vi "PKG_Fill_MUL32A.vi"(1 "dest_axis":i16, 4 "dest":i16, 5 "Src2_axis":i16, 6 "Src2":i16, 7 "Src1_axis":i16, 9 "Src1":i16, 10 "EventType":i16, 11 "info":T1) -> (2 "function return":i32, 3 "info out":T1)   [LabVIEW 2011, in "IMC_Pkg4xxx.lvlib"]
doc: "IMC_PKG_API int WINAPI PKG_Fill_MUL32A(EventInfo *info, short EventType, short Src1, short Src1_axis, short Src2, short Src2_axis, short dest, short dest_axis);\n\n\nIMC_PKG_API int WINAPI PKG_Fill_SCA32(EventInfo *info, short EventType, short Src1, short Src1_axis, short Src2, short Src2_axis, short dest, short dest_axis); IMC_PKG_API int WINAPI PKG_Fill_SCA32i(EventInfo *info, short EventType, short Src1, short Src1_axis, double data, short dest, short dest_axis); IMC_PKG_API int WINAPI PKG_Fill_SCA48(EventInfo *info, short EventType, short Src1, short Src1_axis, short Src2, short Src2_axis, short dest, short dest_axis); IMC_PKG_API int WINAPI PKG_Fill_SCA48i(EventInfo *info, short EventType, short Src1, short Src1_axis, double data, short dest, short dest_axis); IMC_PKG_API int WINAPI PKG_Fill_MUL32L(EventInfo *info, short EventType, short Src1, short Src1_axis, short Src2, short Src2_axis, short dest, short dest_axis); IMC_PKG_API int WINAPI PKG_Fill_MUL32iL(EventInfo *info, short EventType, short Src1, short Src1_axis, long data, short dest, short dest_axis); IMC_PKG_API int WINAPI PKG_Fill_MUL32A(EventInfo *info, short EventType, short Src1, short Src1_axis, short Src2, short Src2_axis, short dest, short dest_axis);"
uses:
  IMC_Pkg4xxx.lvlib
  IMC_Pkg4xxx.dll
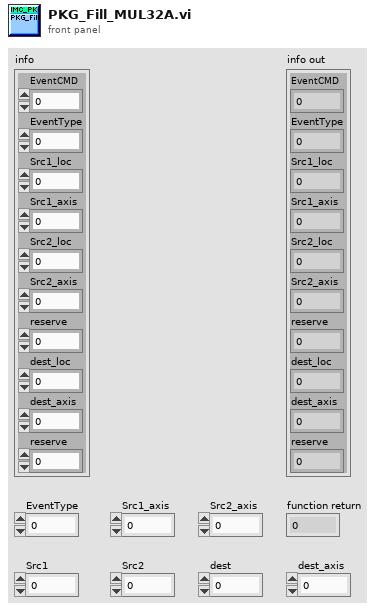
[diagram p1: front panel]
types:
  T1 = cluster{"EventCMD":i16, "EventType":i16, "Src1_loc":i16, "Src1_axis":i16, "Src2_loc":i16, "Src2_axis":i16, "reserve":i32, "dest_loc":i16, "dest_axis":i16, "reserve":i32}
diagram:
  # "IMC_PKG_API int WINAPI PKG_Fill_MUL32A(EventInfo *info, \t\t\t\t\tshort  EventType, \t\t\t\t\t\t\t\t\t\tshort Src1, short Src1_axis, \t\t                    short Src2, short Src2_axis,  \t\t                    short dest, short dest_axis);\n\n\nIMC_PKG_API int WINAPI PKG_Fill_SCA32(EventInfo *info,  \t\t\t\t\tshort  EventType, \t\t\t\t\t\t\t\t\t\tshort Src1, short Src1_axis, \t\t                    short Src2, short Src2_axis,  \t\t                    short dest, short dest_axis);\t\tIMC_PKG_API int WINAPI PKG_Fill_SCA32i(EventInfo *info,  \t\t\t\t\tshort  EventType, \t\t\t\t\t\t\t\t\t\tshort Src1, short Src1_axis, \t\t                    double data, \t\t\t\t\t\t\t                    short dest, short dest_axis);\t\tIMC_PKG_API int WINAPI PKG_Fill_SCA48(EventInfo *info,  \t\t\t\t\tshort  EventType, \t\t\t\t\t\t\t\t\t\tshort Src1, short Src1_axis, \t\t                    short Src2, short Src2_axis,  \t\t                    short dest, short dest_axis);\t\tIMC_PKG_API int WINAPI PKG_Fill_SCA48i(EventInfo *info, \t\t\t\t\tshort  EventType, \t\t\t\t\t\t\t\t\t\tshort Src1, short Src1_axis, \t\t                    double data, \t\t\t\t\t\t                    short dest, short dest_axis);\t\tIMC_PKG_API int WINAPI PKG_Fill_MUL32L(EventInfo *info, \t\t\t\t\tshort  EventType, \t\t\t\t\t\t\t\t\t\tshort Src1, short Src1_axis, \t\t                    short Src2, short Src2_axis,  \t\t                    short dest, short dest_axis);\t\tIMC_PKG_API int WINAPI PKG_Fill_MUL32iL(EventInfo *info,\t\t\t\t\tshort  EventType, \t\t\t\t\t\t\t\t\t\tshort Src1, short Src1_axis, \t\t                    long data, \t\t\t\t\t\t\t                    short dest, short dest_axis);\t\tIMC_PKG_API int WINAPI PKG_Fill_MUL32A(EventInfo *info, \t\t\t\t\tshort  EventType, \t\t\t\t\t\t\t\t\t\tshort Src1, short Src1_axis, \t\t                    short Src2, short Src2_axis,  \t\t                    short dest, short dest_axis);"
  n1 = dll-call lib="PTH1mabs F光盘刻录\niMC MotionIMCNet_V4.0IMCAppincLabviewIMC_PKG4xxxIMC_PKG4xxx\nIMC_Pkg4xxx.*" fn="PKG_Fill_MUL32A"("info"="info", "EventType"="EventType", "Src1"="Src1", "Src1_axis"="Src1_axis", "Src2"="Src2", "Src2_axis"="Src2_axis", "dest"="dest", "dest_axis"="dest_axis") -> (→"function return":i32, "info"=→"info out":T1)  [unwired: 10 in, 2 out]
